vi "leaks.vi"() -> ()   [LabVIEW 2009, in "run.lvlib"]
uses:
  Hal/testing/run.lvlib
  NativeXML.lvclass
panel:
  in  "Path":path=path "C:/Documents and Settings/Administrator/Desktop/Crete/Data/Scripts/Settings Database/DeviceSettingsAtomChip.xml"
  in  "stop":bool
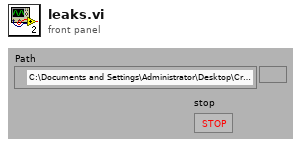
[diagram p1: front panel]
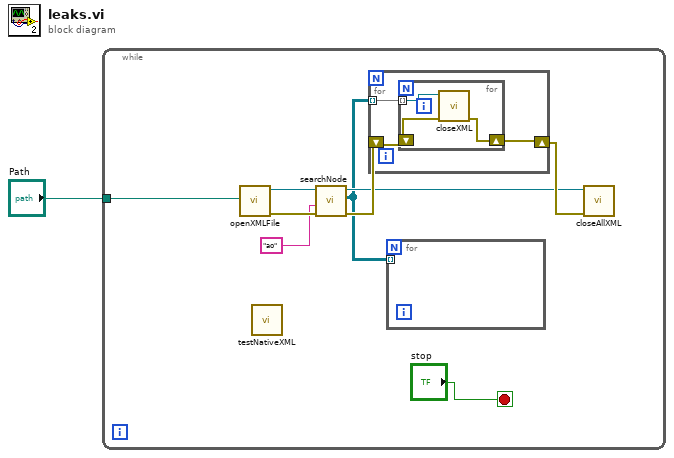
[diagram p0: block diagram]
diagram:
  n1 = while {
    tunnel: "Path" -> [w9]
    stop <- "stop" stop-if-true
    n2 = call "openXMLFile.vi"("Path"=w9) -> ("error out"=w7:errorcluster, "NativeXML out"=w8:refnum<class "NativeXML.lvclass">)  [unwired: 9 in]
    n3 = call "testNativeXML.vi"() -> ()  [unwired: 11 in, 1 out]
    n4 = call "searchNode.vi"("error in (no error)"=w7, "searchElementName"="ao", "NativeXML in"=w8) -> ("error out"=w5:errorcluster, "nodeArray"=w2:refnum<class "NativeXML.lvclass">[][], "NativeXML out"=w3:refnum<class "NativeXML.lvclass">)  [unwired: 6 in]
    n5 = for {
      tunnel: w2 -> [w13] mode=indexing
      shift-right: [w11] -> w4
      shift-left: w5 -> [w12]
      n6 = for {
        tunnel: w13 -> [w16] mode=indexing
        shift-right: [w14] -> w11
        shift-left: w12 -> [w15]
        n7 = call "closeXML.vi"("error in (no error)"=w15, "NativeXML in"=w16) -> ("error out"=w14:errorcluster)  [unwired: 9 in]
      }
    }
    n8 = for {
      tunnel: w2 -> [_] mode=indexing
    }
    n9 = call "closeAllXML.vi"("error in (no error)"=w4, "NativeXML in"=w3) -> ()  [unwired: 9 in, 1 out]
  }
